vi "Update Value Control.vi"(7 "Force update?":bool, 8 "error in (no error)":errorcluster, 9 "Tab Control Ref In":T1, 10 "Tree Control In":refnum<vi>, 11 "Session In":T2) -> (0 "error out":errorcluster, 1 "Units":string, 2 "Tooltip":string, 3 "Session Out":T2)   [LabVIEW 2015, in "CameraSetup.lvlib"]
doc: "The Update Value Control subVI determines the type of the attribute selected, displays the corresponding tab in the tab control, sets the current value of the control, sets the minimum and maximum of the control (for numerics), and disables the control if the attribute is not writables."
uses:
  CameraSetup.lvlib
  <vilib>/userdefined/High Color/IMAQdx.ctl
  <vilib>/vision/driver/IMAQdx.llb/IMAQdx Attribute Type.ctl
  <vilib>/vision/driver/NI_Vision_Acquisition_Software.lvlib
  <resource>/objmgr/imaqdx.rc
panel:
  # "Overview: Demonstrates\nRequirements: Vision Acquisition Software\nInstructions: Run the VI"
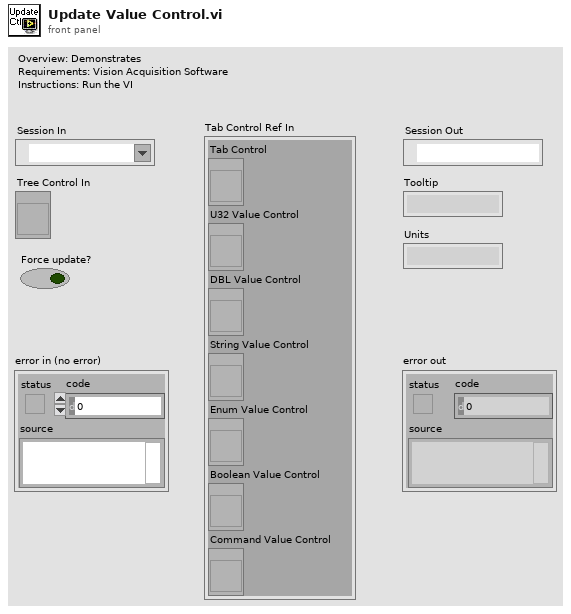
[diagram p1: front panel]
types:
  T1 = cluster{"Tab Control":refnum<vi>, "U32 Value Control":refnum<vi>, "DBL Value Control":refnum<vi>, "String Value Control":refnum<vi>, "Enum Value Control":refnum<vi>, "Boolean Value Control":refnum<vi>, "Command Value Control":refnum<vi>}
  T2 = typedef "IMAQdx.ctl" = refnum<k21>
  T3 = typedef "NI_Vision_Acquisition_Software.lvlib/IMAQdx Attribute Type.ctl" = enum32{"U32", "I64", "DBL", "String", "Enum", "Bool", "Command"}
  T4 = enum32{"U32", "DBL", "String", "Enum", "Bool", "Command"}
  T5 = enum8{"Enabled", "Disabled", "Disabled and Grayed Out"}
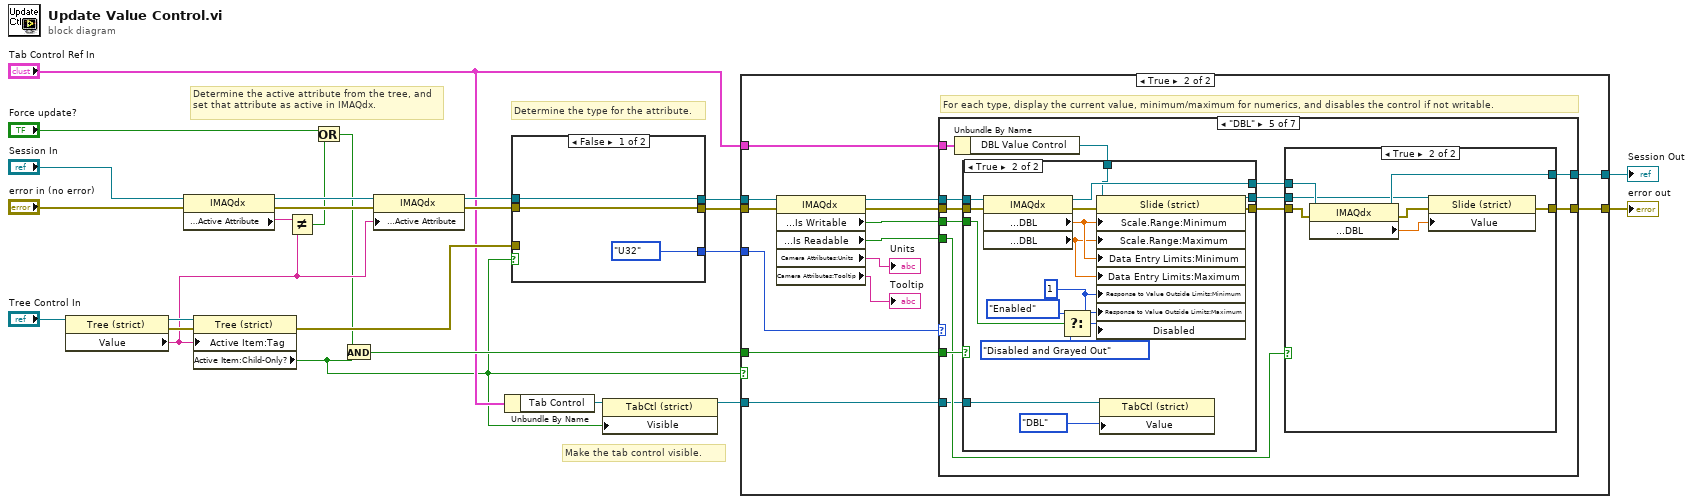
[diagram p0: block diagram]
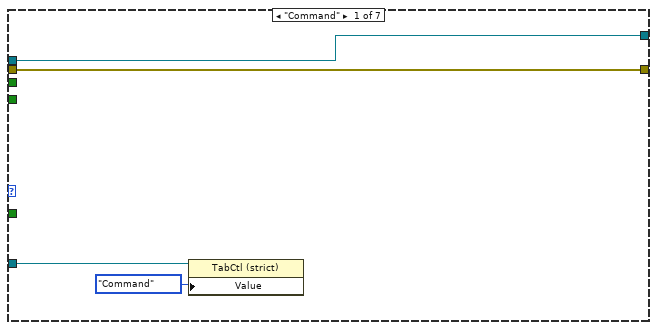
[diagram p3: hidden frame]
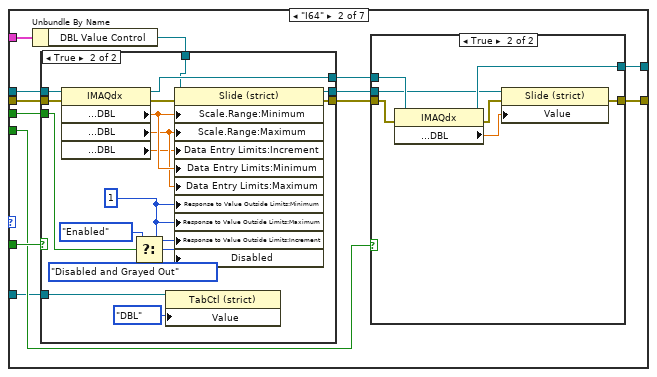
[diagram p4: hidden frame]
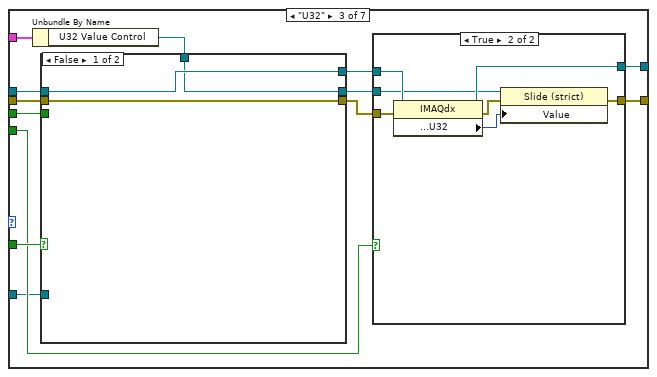
[diagram p7: hidden frame]
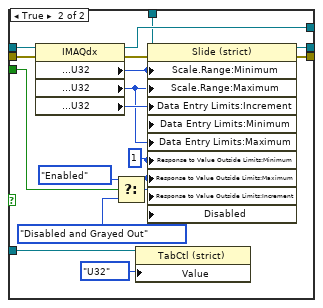
[diagram p9: hidden frame]
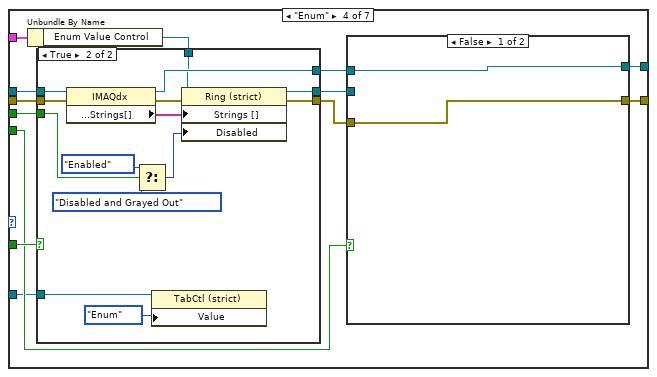
[diagram p10: hidden frame]
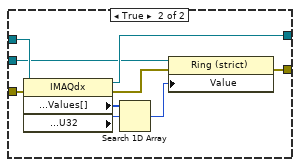
[diagram p11: hidden frame]
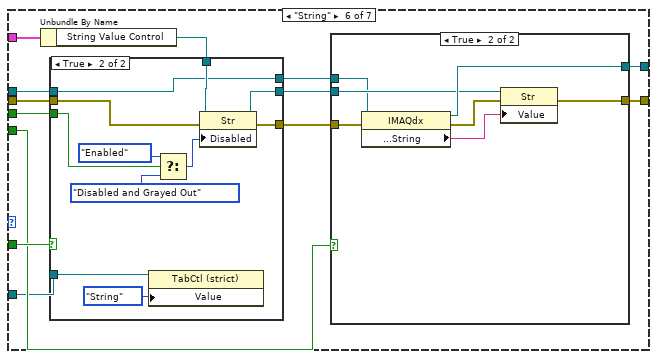
[diagram p15: hidden frame]
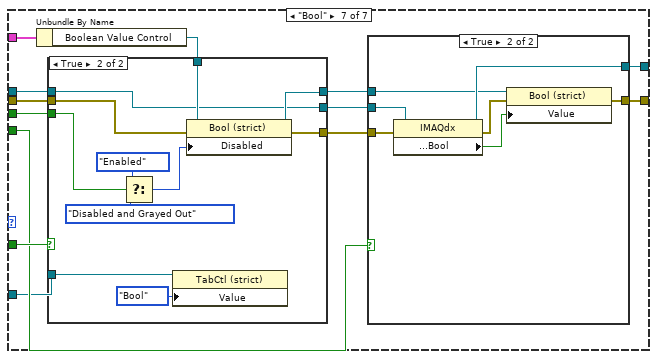
[diagram p18: hidden frame]
diagram:
  # "Make the tab control visible."
  # "Determine the type for the attribute."
  # "Determine the active attribute from the tree, and set that attribute as active in IMAQdx."
  n1 = property class="Tree (strict)"(reference="Tree Control In") -> (reference out=w11:refnum<vi>, error out=w10:errorcluster, "Value"=w9:string)  [unwired: 1 in]
  n2 = property class="IMAQdx"(reference="Session In", error in="error in (no error)") -> (reference out=w24:T2, error out=w23:errorcluster, "Camera Attributes:Active Attribute"=w25:string)
  n3 = property class="Tree (strict)"(reference=w11, error in=w10, "Active Item:Tag"=w9) -> (error out=w16:errorcluster, "Active Item:Child-Only?"=w1:bool)  [unwired: 1 out]
  n4 = Not Equal?(x=w25, y=w9) -> (x != y?=w4:bool)
  n5 = Or(x="Force update?", y=w4) -> (x .or. y?=w2:bool)
  n6 = And(x=w2, y=w1) -> (x .and. y?=w17:bool)
  n7 = property class="IMAQdx"(reference=w24, error in=w23, "Camera Attributes:Active Attribute"=w9) -> (reference out=w22:T2, error out=w21:errorcluster)
  n8 = Unbundle By Name("Tab Control Ref In") -> ("Tab Control"=w7:refnum<vi>)
  n9 = case shown="False" w1 {
    tunnel: w22 -> [w28 w35]
    tunnel: [w28 w32] -> w19
    tunnel: [IMAQdx_Attribute_Type."U32" ("Attribute Type") w31] -> w18
    tunnel: w21 -> [w26 w30]
    tunnel: [w26 w29] -> w20
    tunnel: w16 -> [_ _]
    frame False {
    }
    frame True {
      n10 = property class="IMAQdx"(reference=w35, error in=w30) -> (reference out=w32:T2, error out=w29:errorcluster, "Camera Attributes:Type"=w34:u32)
      n11 = Type Cast(type=IMAQdx_Attribute_Type."U32" ("Attribute Type"), x=w34) -> (*(type *) &x=w31:T3)
    }
  }
  n12 = property class="TabCtl (strict)"(reference=w7, "Visible"=w1) -> (reference out=w5:refnum<vi>)  [unwired: 1 in, 1 out]
  n13 = case shown="True" w1 {
    tunnel: w20 -> [w37 w50]
    tunnel: [w37 w43] -> w12
    tunnel: w19 -> [w36 w51]
    tunnel: w18 -> [_ w48]
    tunnel: w17 -> [_ w38]
    tunnel: [w36 w42] -> w13
    tunnel: "Tab Control Ref In" -> [_ w41]
    tunnel: w5 -> [_ w40]
    frame False {
    }
    frame True {
      # "For each type, display the current value, minimum/maximum for numerics, and disables the control if not writable."
      n14 = property class="IMAQdx"(reference=w51, error in=w50) -> (reference out=w45:T2, error out=w44:errorcluster, "Camera Attributes:Is Writable"=w47:bool, "Camera Attributes:Is Readable"=w46:bool, "Camera Attributes:Units"=→"Units":string, "Camera Attributes:Tooltip"=→"Tooltip":string)
      n15 = case shown="\"DBL\"" w48 {
        tunnel: w47 -> [_ w65 w107 w149 w190 w231 w267]
        tunnel: w46 -> [_ w64 w106 w148 w189 w230 w266]
        tunnel: w45 -> [w54 w68 w110 w152 w193 w234 w270]
        tunnel: w44 -> [w55 w67 w109 w151 w192 w233 w269]
        tunnel: w38 -> [_ w66 w108 w150 w191 w232 w268]
        tunnel: [w55 w61 w103 w146 w186 w228 w264] -> w43
        tunnel: [w54 w60 w102 w145 w185 w227 w263] -> w42
        tunnel: w41 -> [_ w58 w99 w142 w184 w225 w261]
        tunnel: w40 -> [w53 w59 w100 w143 w182 w226 w262]
        frame "Command" {
          n16 = property class="TabCtl (strict)"(reference=w53, "Value"=T4."Command" ("Tab Control")) -> ()  [unwired: 1 in, 2 out]
        }
        frame "I64" {
          n17 = Unbundle By Name(w58) -> ("DBL Value Control"=w57:refnum<vi>)
          n18 = case shown="True" w66 {
            tunnel: w68 -> [w80 w97]
            tunnel: w67 -> [w79 w96]
            tunnel: [w80 w92] -> w63
            tunnel: [w79 w88] -> w62
            tunnel: w65 -> [_ w95]
            tunnel: w59 -> [_ w94]
            tunnel: w57 -> [w78 w90]
            tunnel: [w78 w89] -> w56
            frame False {
            }
            frame True {
              w84 = u8 1 ("Out Of Range Action:Maximum")
              n19 = property class="IMAQdx"(reference=w97, error in=w96) -> (reference out=w92:T2, error out=w91:errorcluster, "Camera Attributes:Minimum:DBL"=w86:dbl, "Camera Attributes:Maximum:DBL"=w85:dbl, "Camera Attributes:Increment:DBL"=w83:dbl)
              n20 = Select(t=T5."Enabled" ("Disabled"), s=w95, f=T5."Disabled and Grayed Out" ("Disabled")) -> (s? t:f=w87:T5)
              n21 = property class="TabCtl (strict)"(reference=w94, "Value"=T4."DBL" ("Tab Control")) -> ()  [unwired: 1 in, 2 out]
              n22 = property class="Slide (strict)"(reference=w90, error in=w91, "Scale.Range:Minimum"=w86, "Scale.Range:Maximum"=w85, "Data Entry Limits:Increment"=w83, "Data Entry Limits:Minimum"=w86, "Data Entry Limits:Maximum"=w85, "Response to Value Outside Limits:Minimum"=w84, "Response to Value Outside Limits:Maximum"=w84, "Response to Value Outside Limits:Increment"=w84, "Disabled"=w87) -> (reference out=w89:refnum<vi>, error out=w88:errorcluster)
            }
          }
          n23 = case shown="True" w64 {
            tunnel: w63 -> [w70 w77]
            tunnel: w62 -> [w69 w76]
            tunnel: [w70 w74] -> w60
            tunnel: [w69 w75] -> w61
            tunnel: w56 -> [_ w72]
            frame False {
            }
            frame True {
              n24 = property class="IMAQdx"(reference=w77, error in=w76) -> (reference out=w74:T2, error out=w73:errorcluster, "Camera Attributes:Value:DBL"=w71:dbl)
              n25 = property class="Slide (strict)"(reference=w72, error in=w73, "Value"=w71) -> (error out=w75:errorcluster)  [unwired: 1 out]
            }
          }
        }
        frame "U32" {
          n26 = Unbundle By Name(w99) -> ("U32 Value Control"=w98:refnum<vi>)
          n27 = case shown="False" w108 {
            tunnel: w110 -> [w122 w139]
            tunnel: w109 -> [w121 w138]
            tunnel: [w122 w135] -> w105
            tunnel: [w121 w133] -> w104
            tunnel: w107 -> [_ w137]
            tunnel: [w120 w132] -> w101
            tunnel: w100 -> [_ w131]
            tunnel: w98 -> [w120 w129]
            frame False {
            }
            frame True {
              w128 = u8 1 ("Out Of Range Action:Maximum")
              n28 = property class="IMAQdx"(reference=w139, error in=w138) -> (reference out=w135:T2, error out=w136:errorcluster, "Camera Attributes:Minimum:U32"=w126:u32, "Camera Attributes:Maximum:U32"=w125:u32, "Camera Attributes:Increment:U32"=w127:u32)
              n29 = Select(t=T5."Enabled" ("Disabled"), s=w137, f=T5."Disabled and Grayed Out" ("Disabled")) -> (s? t:f=w134:T5)
              n30 = property class="TabCtl (strict)"(reference=w131, "Value"=T4."U32" ("Tab Control")) -> ()  [unwired: 1 in, 2 out]
              n31 = property class="Slide (strict)"(reference=w129, error in=w136, "Scale.Range:Minimum"=w126, "Scale.Range:Maximum"=w125, "Data Entry Limits:Increment"=w127, "Data Entry Limits:Minimum"=w126, "Data Entry Limits:Maximum"=w125, "Response to Value Outside Limits:Minimum"=w128, "Response to Value Outside Limits:Maximum"=w128, "Response to Value Outside Limits:Increment"=w128, "Disabled"=w134) -> (reference out=w132:refnum<vi>, error out=w133:errorcluster)
            }
          }
          n32 = case shown="True" w106 {
            tunnel: w105 -> [w112 w119]
            tunnel: w104 -> [w111 w118]
            tunnel: [w112 w117] -> w102
            tunnel: [w111 w113] -> w103
            tunnel: w101 -> [_ w114]
            frame False {
            }
            frame True {
              n33 = property class="IMAQdx"(reference=w119, error in=w118) -> (reference out=w117:T2, error out=w116:errorcluster, "Camera Attributes:Value:U32"=w115:u32)
              n34 = property class="Slide (strict)"(reference=w114, error in=w116, "Value"=w115) -> (error out=w113:errorcluster)  [unwired: 1 out]
            }
          }
        }
        frame "Enum" {
          n35 = Unbundle By Name(w142) -> ("Enum Value Control"=w141:refnum<vi>)
          n36 = case shown="True" w150 {
            tunnel: w152 -> [w166 w180]
            tunnel: w151 -> [w165 w179]
            tunnel: [w166 w177] -> w147
            tunnel: [w165 w175] -> w140
            tunnel: w149 -> [_ w178]
            tunnel: [w164 w174] -> w144
            tunnel: w143 -> [_ w171]
            tunnel: w141 -> [w164 w169]
            frame False {
            }
            frame True {
              n37 = property class="IMAQdx"(reference=w180, error in=w179) -> (reference out=w177:T2, error out=w176:errorcluster, "Camera Attributes:Enum:Strings[]"=w172:string[])
              n38 = Select(t=T5."Enabled" ("Disabled"), s=w178, f=T5."Disabled and Grayed Out" ("Disabled")) -> (s? t:f=w173:T5)
              n39 = property class="TabCtl (strict)"(reference=w171, "Value"=T4."Enum" ("Tab Control")) -> ()  [unwired: 1 in, 2 out]
              n40 = property class="Ring (strict)"(reference=w169, error in=w176, "Strings []"=w172, "Disabled"=w173) -> (reference out=w174:refnum<vi>, error out=w175:errorcluster)
            }
          }
          n41 = case shown="False" w148 {
            tunnel: w147 -> [w154 w163]
            tunnel: [w154 w158] -> w145
            tunnel: [w153 w160] -> w146
            tunnel: w144 -> [_ w157]
            tunnel: w140 -> [w153 w155]
            frame False {
            }
            frame True {
              n42 = property class="IMAQdx"(reference=w163, error in=w155) -> (reference out=w158:T2, error out=w156:errorcluster, "Camera Attributes:Enum:Values[]"=w162:u32[], "Camera Attributes:Value:U32"=w161:u32)
              n43 = Search 1D Array(1D array=w162, element=w161) -> (index of element=w159:i32)  [unwired: 1 out]
              n44 = property class="Ring (strict)"(reference=w157, error in=w156, "Value"=w159) -> (error out=w160:errorcluster)  [unwired: 1 out]
            }
          }
        }
        frame "DBL" {
          n45 = Unbundle By Name(w184) -> ("DBL Value Control"=w183:refnum<vi>)
          n46 = case shown="True" w191 {
            tunnel: w193 -> [w205 w221]
            tunnel: w192 -> [w204 w220]
            tunnel: [w205 w218] -> w188
            tunnel: [w204 w213] -> w187
            tunnel: w190 -> [_ w219]
            tunnel: w183 -> [w203 w216]
            tunnel: [w203 w215] -> w181
            tunnel: w182 -> [_ w212]
            frame False {
            }
            frame True {
              w206 = u8 1 ("Out Of Range Action:Minimum")
              n47 = property class="IMAQdx"(reference=w221, error in=w220) -> (reference out=w218:T2, error out=w217:errorcluster, "Camera Attributes:Minimum:DBL"=w210:dbl, "Camera Attributes:Maximum:DBL"=w209:dbl)
              n48 = Select(t=T5."Enabled" ("Disabled"), s=w219, f=T5."Disabled and Grayed Out" ("Disabled")) -> (s? t:f=w214:T5)
              n49 = property class="Slide (strict)"(reference=w216, error in=w217, "Scale.Range:Minimum"=w210, "Scale.Range:Maximum"=w209, "Data Entry Limits:Minimum"=w210, "Data Entry Limits:Maximum"=w209, "Response to Value Outside Limits:Minimum"=w206, "Response to Value Outside Limits:Maximum"=w206, "Disabled"=w214) -> (reference out=w215:refnum<vi>, error out=w213:errorcluster)
              n50 = property class="TabCtl (strict)"(reference=w212, "Value"=T4."DBL" ("Tab Control")) -> ()  [unwired: 1 in, 2 out]
            }
          }
          n51 = case shown="True" w189 {
            tunnel: w188 -> [w195 w202]
            tunnel: w187 -> [w194 w201]
            tunnel: [w195 w200] -> w185
            tunnel: [w194 w198] -> w186
            tunnel: w181 -> [_ w197]
            frame False {
            }
            frame True {
              n52 = property class="IMAQdx"(reference=w202, error in=w201) -> (reference out=w200:T2, error out=w199:errorcluster, "Camera Attributes:Value:DBL"=w196:dbl)
              n53 = property class="Slide (strict)"(reference=w197, error in=w199, "Value"=w196) -> (error out=w198:errorcluster)  [unwired: 1 out]
            }
          }
        }
        frame "String" {
          n54 = Unbundle By Name(w225) -> ("String Value Control"=w224:refnum<vi>)
          n55 = case shown="True" w232 {
            tunnel: w234 -> [w244 w249]
            tunnel: w233 -> [w246 w253]
            tunnel: [w246 w252] -> w229
            tunnel: w231 -> [_ w257]
            tunnel: w226 -> [_ w256]
            tunnel: w224 -> [w245 w254]
            tunnel: [w245 w250] -> w223
            tunnel: [w244 w249] -> w222
            frame False {
            }
            frame True {
              n56 = property class="TabCtl (strict)"(reference=w256, "Value"=T4."String" ("Tab Control")) -> ()  [unwired: 1 in, 2 out]
              n57 = Select(t=T5."Enabled" ("Disabled"), s=w257, f=T5."Disabled and Grayed Out" ("Disabled")) -> (s? t:f=w251:T5)
              n58 = property class="Str"(reference=w254, error in=w253, "Disabled"=w251) -> (reference out=w250:refnum<vi>, error out=w252:errorcluster)
            }
          }
          n59 = case shown="True" w230 {
            tunnel: w229 -> [w236 w243]
            tunnel: [w235 w242] -> w227
            tunnel: [w236 w240] -> w228
            tunnel: w223 -> [_ w238]
            tunnel: w222 -> [w235 w237]
            frame False {
            }
            frame True {
              n60 = property class="IMAQdx"(reference=w237, error in=w243) -> (reference out=w242:T2, error out=w241:errorcluster, "Camera Attributes:Value:String"=w239:string)
              n61 = property class="Str"(reference=w238, error in=w241, "Value"=w239) -> (error out=w240:errorcluster)  [unwired: 1 out]
            }
          }
        }
        frame "Bool" {
          n62 = Unbundle By Name(w261) -> ("Boolean Value Control"=w260:refnum<vi>)
          n63 = case shown="True" w268 {
            tunnel: w270 -> [w280 w285]
            tunnel: w269 -> [w282 w288]
            tunnel: [w282 w287] -> w265
            tunnel: w267 -> [_ w293]
            tunnel: w262 -> [_ w292]
            tunnel: w260 -> [w281 w290]
            tunnel: [w281 w289] -> w259
            tunnel: [w280 w285] -> w258
            frame False {
            }
            frame True {
              n64 = Select(t=T5."Enabled" ("Disabled"), s=w293, f=T5."Disabled and Grayed Out" ("Disabled")) -> (s? t:f=w286:T5)
              n65 = property class="TabCtl (strict)"(reference=w292, "Value"=T4."Bool" ("Tab Control")) -> ()  [unwired: 1 in, 2 out]
              n66 = property class="Bool (strict)"(reference=w290, error in=w288, "Disabled"=w286) -> (reference out=w289:refnum<vi>, error out=w287:errorcluster)
            }
          }
          n67 = case shown="True" w266 {
            tunnel: w265 -> [w272 w279]
            tunnel: [w271 w278] -> w263
            tunnel: [w272 w276] -> w264
            tunnel: w259 -> [_ w274]
            tunnel: w258 -> [w271 w273]
            frame False {
            }
            frame True {
              n68 = property class="IMAQdx"(reference=w273, error in=w279) -> (reference out=w278:T2, error out=w277:errorcluster, "Camera Attributes:Value:Bool"=w275:bool)
              n69 = property class="Bool (strict)"(reference=w274, error in=w277, "Value"=w275) -> (error out=w276:errorcluster)  [unwired: 1 out]
            }
          }
        }
      }
    }
  }
  "Session Out" <- w13
  "error out" <- w12
